vi "Handle Messages.vi"(8 "error in (no error)":errorcluster, 9 "Message Data":variant, 10 "Message":string, 11 "Customer In":refnum<class "Customer.lvclass">) -> (0 "error out":errorcluster, 3 "Customer Out":refnum<class "Customer.lvclass">)   [LabVIEW 2020, in "Customer.lvclass"]
uses:
  Customer.lvclass
  Support/Beverages/Beverage/Beverage.lvclass
  Customer.lvclass/Customer.ctl
  Person/Person.lvclass
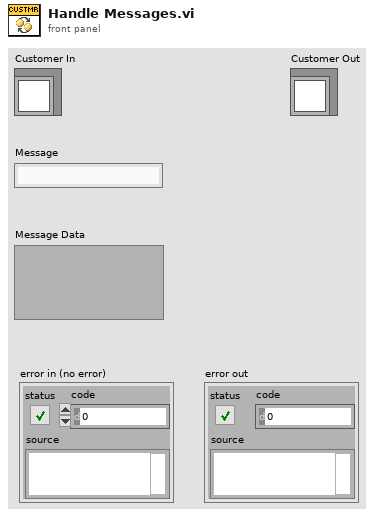
[diagram p1: front panel]
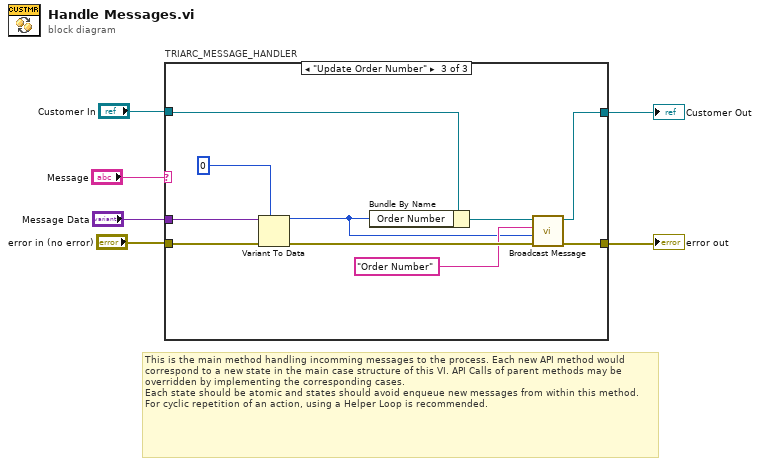
[diagram p0: block diagram]
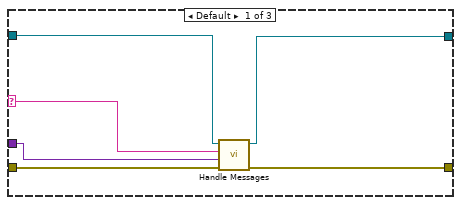
[diagram p2: hidden frame]
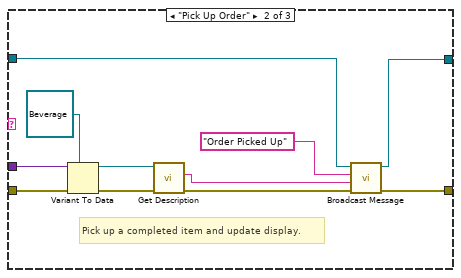
[diagram p3: hidden frame]
diagram:
  # "This is the main method handling incomming messages to the process. Each new API method would correspond to a new state in the main case structure of this VI. API Calls of parent methods may be overridden by implementing the corresponding cases.\nEach state should be atomic and states should avoid enqueue new messages from within this method. For cyclic repetition of an action, using a Helper Loop is recommended."
  n1 = case "TRIARC_MESSAGE_HANDLER" shown="\"Update Order Number\"" "Message" {
    selector: "Message" -> [w10 _ _]
    tunnel: "error in (no error)" -> [w9 w23 w33]
    tunnel: "Customer In" -> [w12 w21 w28]
    tunnel: "Message Data" -> [w11 w19 w31]
    tunnel: [w8 w22 w29] -> w2
    tunnel: [w7 w20 w26] -> w1
    frame Default {
      n2 = call-parent "Handle Messages.vi"("error in (no error)"=w9, "Message Data"=w11, "Message"=w10, "Person In"=w12) -> ("error out"=w8:errorcluster, "Person Out"=w7:refnum<class "Customer.lvclass">)  [unwired: 6 in]
    }
    frame "Pick Up Order" {
      # "Pick up a completed item and update display."
      n3 = Variant To Data(error in=w23, type=refnum<class "Beverage.lvclass"> refnum ("Beverage.lvclass"), Variant=w19) -> (data=w16:refnum<class "Beverage.lvclass">, error out=w15:errorcluster)
      n4 = call "Get Description.vi"("error in"=w15, "Beverage in"=w16) -> ("error out"=w14:errorcluster, "Description"=w13:string)  [unwired: 7 in, 1 out]
      n5 = call-dynamic "Broadcast Message.vi"("error in (no error)"=w14, "Message Data"=w13, "Message"="Order Picked Up", "Rig Process In"=w21) -> ("error out"=w22:errorcluster, "Rig Process Out"=w20:refnum<class "Customer.lvclass">)  [unwired: 6 in]
    }
    frame "Update Order Number" {
      n6 = Variant To Data(error in=w33, type=u32 0 ("Order Number"), Variant=w31) -> (data=w24:u32, error out=w32:errorcluster)
      n7 = Bundle By Name(cluster=w28, "Order Number"=w24) -> (w27:refnum<class "Customer.lvclass">)
      n8 = call-dynamic "Broadcast Message.vi"("error in (no error)"=w32, "Message Data"=w24, "Message"="Order Number", "Rig Process In"=w27) -> ("error out"=w29:errorcluster, "Rig Process Out"=w26:refnum<class "Customer.lvclass">)  [unwired: 6 in]
    }
  }
  "error out" <- w2
  "Customer Out" <- w1
